vi "Exit.vi"(8 "error in":errorcluster, 10 "Message Queues":T2, 11 "Notifiers":T1) -> (0 "error out":errorcluster)   [LabVIEW 2014, in "Logger.lvlib"]
uses:
  Logger.lvlib
  support/Message Queue/Message Queue.lvlib
  support/Message Queue/Message Cluster.ctl
  support/Message Queue/All Message Queues.ctl
  support/Notifiers/Notifiers.ctl
  Support/Notifiers/Notifiers.lvlib
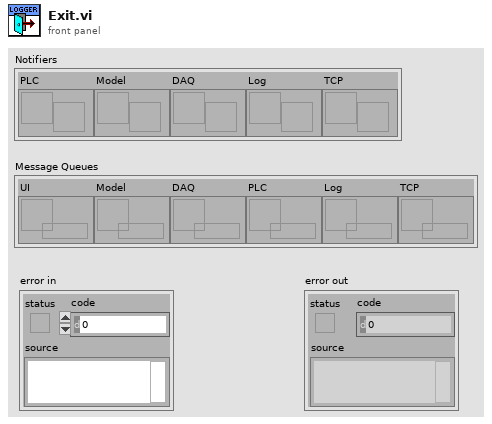
[diagram p1: front panel]
types:
  T1 = typedef "Notifiers.lvlib/Notifiers.ctl" = cluster{"PLC":refnum<notifier>, "Model":refnum<notifier>, "DAQ":refnum<notifier>, "Log":refnum<notifier>, "TCP":refnum<notifier>}
  T2 = typedef "Message Queue.lvlib/All Message Queues.ctl" = cluster{"UI":refnum<queue>, "Model":refnum<queue>, "DAQ":refnum<queue>, "PLC":refnum<queue>, "Log":refnum<queue>, "TCP":refnum<queue>}
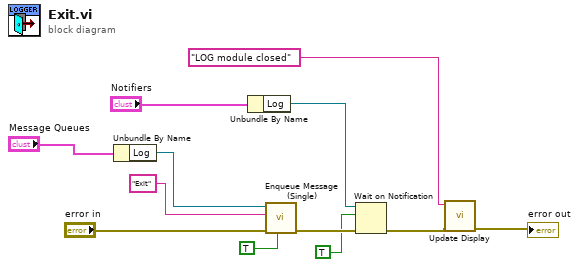
[diagram p0: block diagram]
diagram:
  n1 = Unbundle By Name("Message Queues") -> ("Log"=w5:refnum<queue>)
  n2 = Unbundle By Name("Notifiers") -> ("Log"=w6:refnum<notifier>)
  n3 = call "Enqueue Message (Single).vi"("Priority Message? (F)"=TRUE, "error in (no error)"="error in", "Message"="Exit", "Message Queue"=w5) -> ("error out"=w10:errorcluster)  [unwired: 6 in, 1 out]
  n4 = Wait on Notification(notifier=w6, ignore previous (F)=TRUE, error in (no error)=w10) -> (error out=w4:errorcluster)  [unwired: 1 in, 3 out]
  n5 = call "Update Display.vi"("error in"=w4, "Message string"="LOG module closed" ("Message")) -> ("error out"=→"error out":errorcluster)  [unwired: 9 in]
